vi "PWM CAP Get Data.vi"(9 "pPWMData":cluster{"LowValue":u16, "HighValue":u16}, 10 "Channel":u8, 11 "DevHandle":i32) -> (1 "pPWMData out":cluster{"LowValue":u16, "HighValue":u16}, 3 "function return":i32)   [LabVIEW 2010, in "usb2pwm.lvlib"]
doc: "int WINAPI PWM_CAP_GetData(int DevHandle, unsigned char Channel,PWM_CAP_DATA *pPWMData);"
uses:
  usb2pwm.lvlib
  USB2XXX/trunk/USB2XXX/USB2XXX/vs2019/Release/USB2XXX.dll
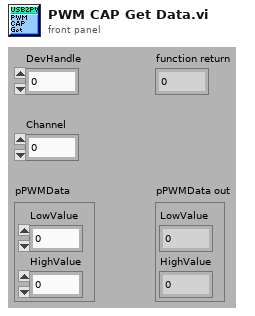
[diagram p1: front panel]
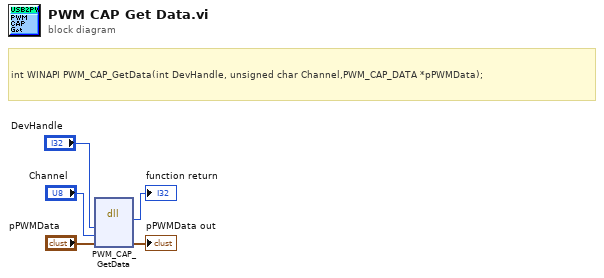
[diagram p0: block diagram]
diagram:
  # "int WINAPI PWM_CAP_GetData(int DevHandle, unsigned char Channel,PWM_CAP_DATA *pPWMData);"
  n1 = dll-call lib="E:/Projects/USB2XXX/trunk/USB2XXX/USB2XXX/vs2019/Release/USB2XXX.*" fn="PWM_CAP_GetData"("DevHandle"="DevHandle", "Channel"="Channel", "pPWMData"="pPWMData") -> (→"function return":i32, "pPWMData"=→"pPWMData out":cluster{"LowValue":u16, "HighValue":u16})  [unwired: 5 in, 2 out]
